vi "Get VI By ID.vi"(8 "error in (no error)":errorcluster, 10 "ID":i32, 11 "Data Cluster in":T1) -> (0 "error out":errorcluster, 2 "VI Reference":refnum<vi>, 3 "Data Cluster out":T1)   [LabVIEW 2025, in "Scripting Server.lvlib"]
uses:
  Scripting Server.lvlib
  Module Data--cluster.ctl
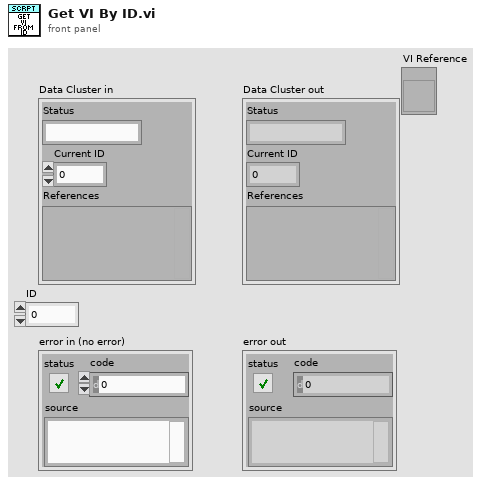
[diagram p1: front panel]
types:
  T1 = typedef "Scripting Server.lvlib/Module Data--cluster.ctl" = cluster{"Status":string, "Current ID":i32, "References":variant}
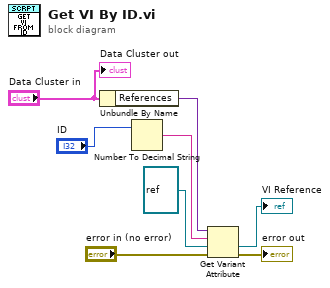
[diagram p0: block diagram]
diagram:
  n1 = Unbundle By Name("Data Cluster in") -> ("References"=w6:variant)
  n2 = Number To Decimal String(number="ID") -> (decimal integer string=w7:string)  [unwired: 1 in]
  n3 = Get Variant Attribute(Variant=w6, name=w7, default value (empty Variant)=refnum<vi> refnum ("vi reference"), error in="error in (no error)") -> (value=→"VI Reference":refnum<vi>, error out=→"error out":errorcluster)  [unwired: 2 out]
  "Data Cluster out" <- "Data Cluster in"
